vi "9_GuessingGame_Template.vi"() -> ()   [LabVIEW 2015]
panel:
  out "message":string
  out "Number of guesses so far":i32
  out "Correct!":bool
  in  "guess":bool
  in  "Number to guess (1-100)":i32
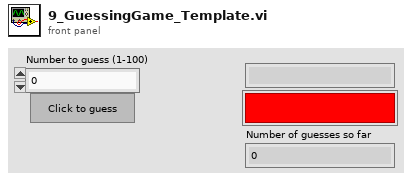
[diagram p1: front panel]
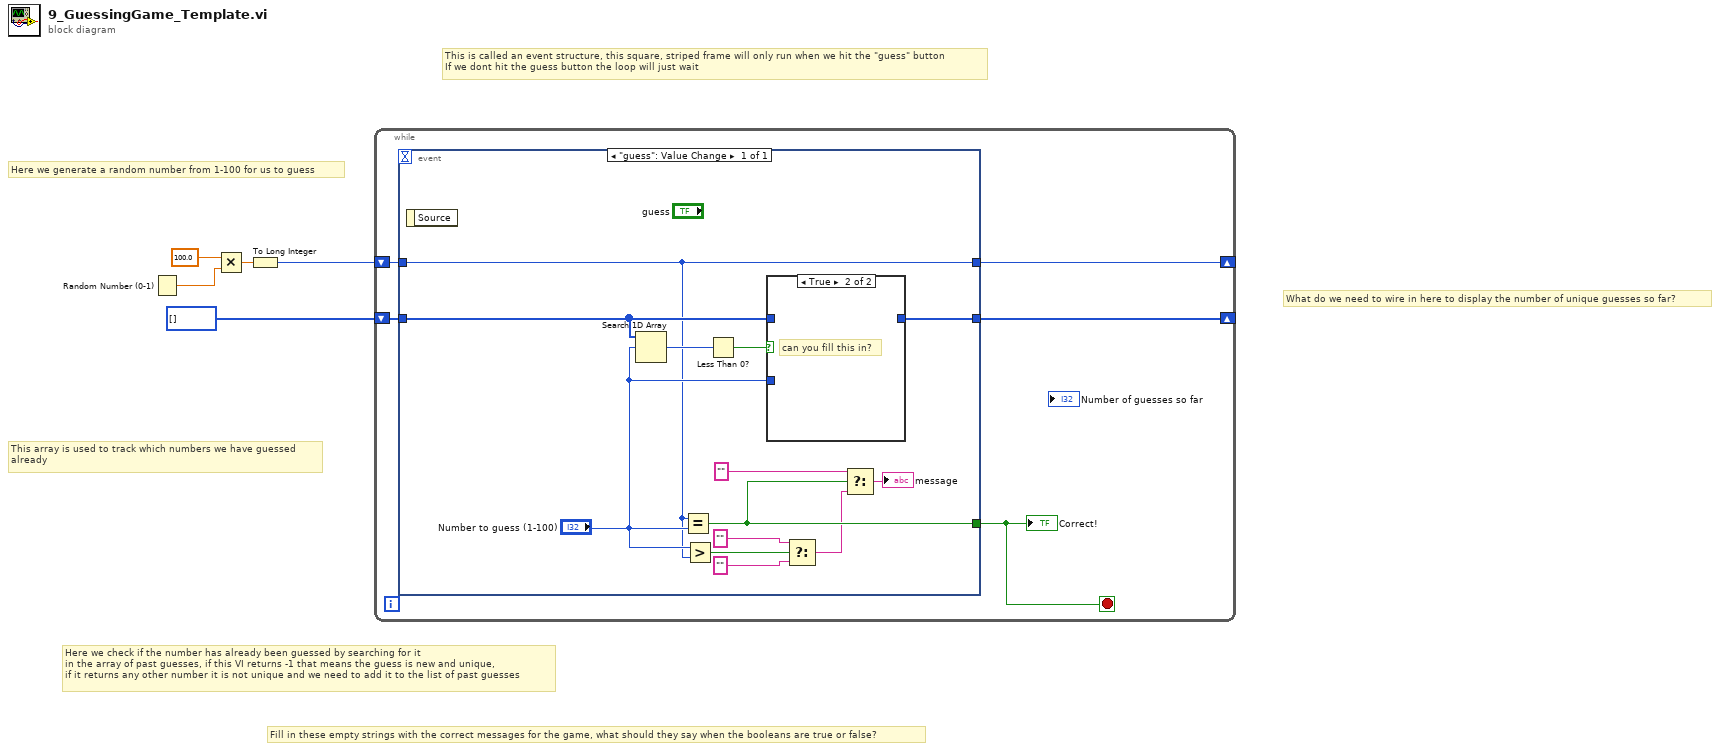
[diagram p0: block diagram]
diagram:
  # "Here we check if the number has already been guessed by searching for it\nin the array of past guesses, if this VI returns -1 that means the guess is new and unique, \nif it returns any other number it is not unique and we need to add it to the list of past guesses"
  # "What do we need to wire in here to display the number of unique guesses so far?"
  # "Here we generate a random number from 1-100 for us to guess"
  # "This array is used to track which numbers we have guessed\nalready"
  # "This is called an event structure, this square, striped frame will only run when we hit the \"guess\" button\nIf we dont hit the guess button the loop will just wait"
  # "Fill in these empty strings with the correct messages for the game, what should they say when the booleans are true or false?"
  n1 = Random Number (0-1)() -> (number: 0 to 1=w4:dbl)
  n2 = Multiply(x=100.0, y=w4) -> (x*y=w3:dbl)
  n3 = To Long Integer(number=w3) -> (32bit integer=w2:i32)
  n4 = while {
    shift-right: [w7] -> _
    shift-left: w2 -> [w9]
    shift-right: [w6] -> _
    shift-left: i32[] [] -> [w8]
    stop <- w10 stop-if-true
    n5 = event shown="[0] \"guess\": Value Change" {
      selector: _ -> [_]
      dyn-events: _ -> [_]
      timeout: _ -> [_]
      tunnel: [w23] -> w10
      tunnel: w9 -> [w15]
      tunnel: w8 -> [w18]
      tunnel: [w15] -> w7
      tunnel: [w17] -> w6
      event "guess": Value Change {
        n6 = event-data() -> ()  [unwired: 1 in, 1 out]
        n7 = Search 1D Array(1D array=w18, element="Number to guess (1-100)") -> (index of element=w20:i32)  [unwired: 1 in]
        n8 = Equal?(x=w15, y="Number to guess (1-100)") -> (x = y?=w23:bool)
        n9 = Greater?(x="Number to guess (1-100)", y=w15) -> (0:w14:bool)
        n10 = Less Than 0?(x=w20) -> (x < 0?=w19:bool)
        n11 = case shown="True" w19 {
          tunnel: w18 -> [w24 _]
          tunnel: "Number to guess (1-100)" -> [_ _]
          tunnel: [w24 _] -> w17
          frame False {
          }
          frame True {
            # "can you fill this in?"
          }
        }
        n12 = Select(t="", s=w14, f="") -> (s? t:f=w11:string)
        n13 = Select(t="", s=w23, f=w11) -> (s? t:f=→"message":string)
      }
    }
    "Correct!" <- w10
  }
